vi "ARCO Instructor Write Client.vi"() -> ()   [LabVIEW 2017]
uses:
  <vilib>/OPCUA/controls/Write Status.ctl
  <vilib>/OPCUA/controls/NodeId.ctl
  <vilib>/OPCUA/client/Multiple Write Double Array.vi
  <vilib>/OPCUA/client/Multiple Write Bool Array.vi
  <vilib>/OPCUA/NI OPC UA Client.lvlib
panel:
  in  "Stop Broadcasting":bool
  in  "Time Stamp":timestamp
  in  "Node Status":T1 items=["Good"=0, "Uncertain_InitialValue"=1083310080, "Uncertain_LastUsableValue"=1083179008, "Uncertain_SensorNotAccurate"=1083375616, "Uncertain_EngineeringUnitsExceeded"=1083441152, "Bad_NoCommunication"=2150694912, "Bad_NotReadable"=2151284736, "Bad_NotWritable"=2151350272, "Bad_OutOfRange"=2151415808, "Bad_WaitingForInitialData"=2150760448]
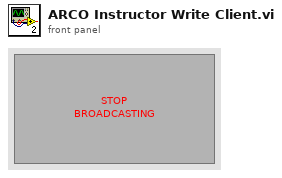
[diagram p1: front panel]
types:
  T1 = typedef "Write Status.ctl" = u32
  T2 = cluster{"message mode":enum16{"None", "Sign", "Sign and Encrypt"}, "security":enum16{"Basic256", "Basic128Rsa15"}}
  T3 = typedef "OPC UA Client Refnum.ctl" = refnum<k21>
  T4 = typedef "NodeId.ctl" = string
  T5 = cluster{"node ID":T4, "value":bool[], "timestamp (current time)":timestamp, "node status":T1}
  T6 = cluster{"node ID":T4, "value":dbl[], "timestamp (current time)":timestamp, "node status":T1}
  T7 = cluster{"node ID":T4, "value":dbl[], "timestamp (current time)":timestamp, "node status":T1}[]
  T8 = cluster{"node ID":T4, "value":bool[], "timestamp (current time)":timestamp, "node status":T1}[]
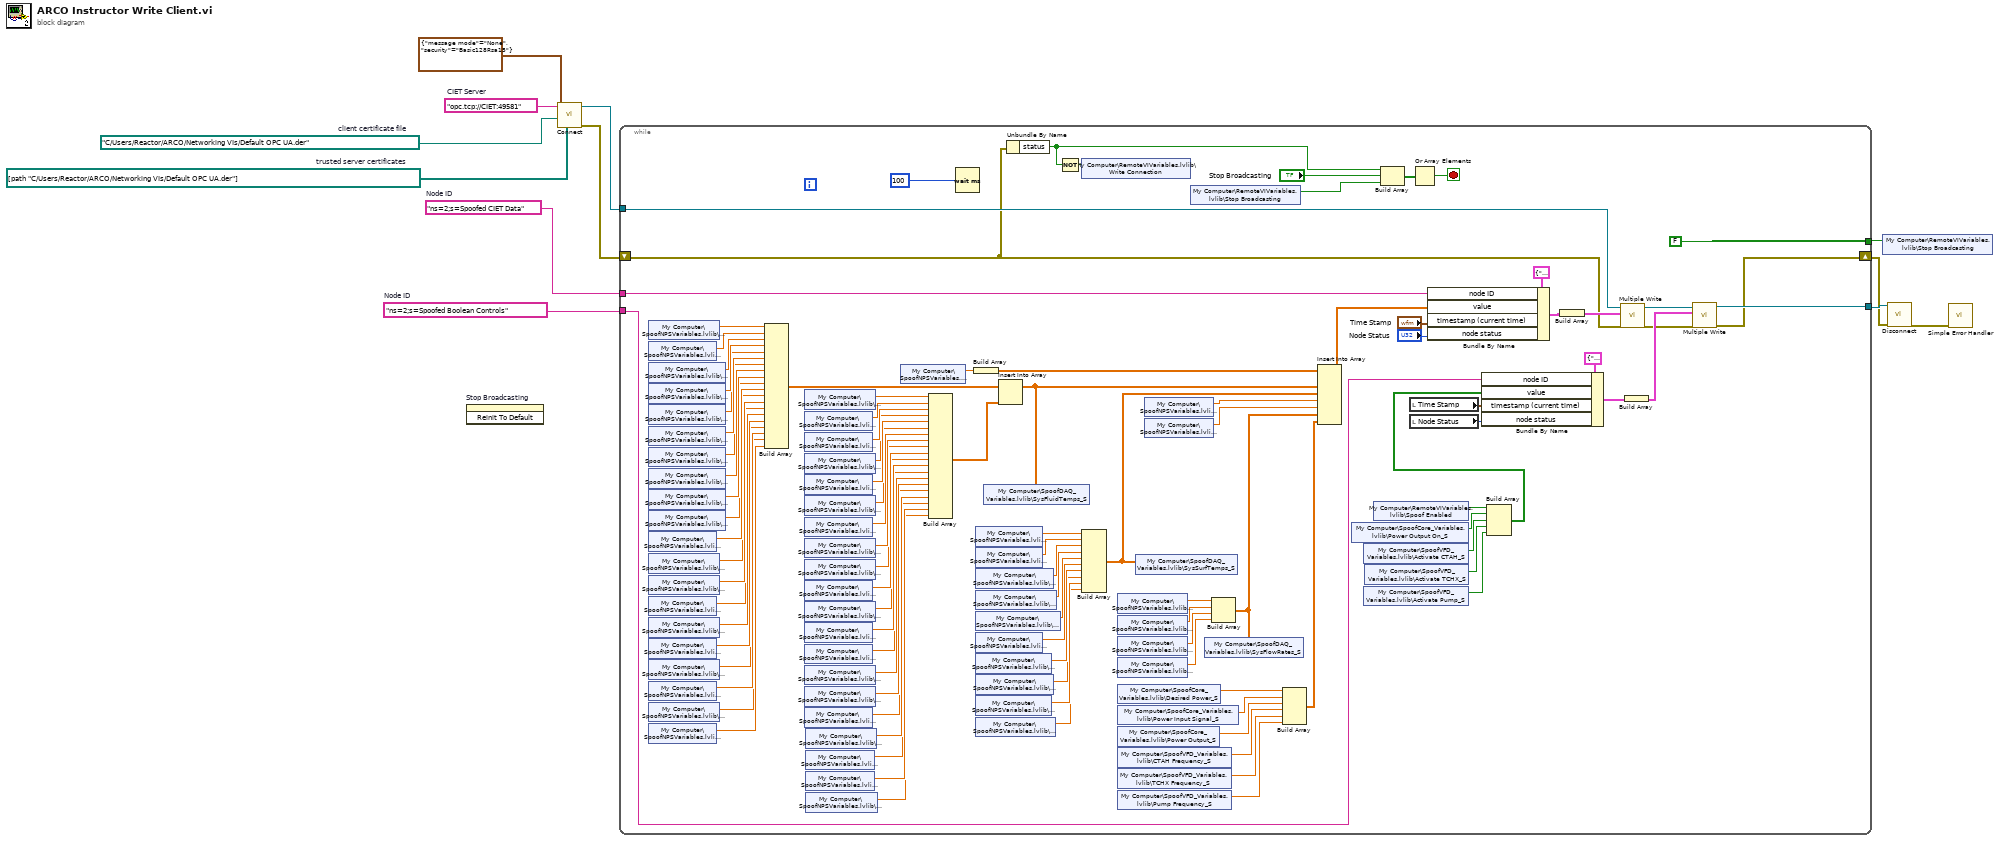
[diagram p0: block diagram]
diagram:
  w1 = "ns=2;s=Spoofed Boolean Controls"  # Node ID
  w6 = path[] [path "C:/Users/Reactor/ARCO/Networking VIs/Default OPC UA.der"]  # trusted server certificates
  w7 = path "C:/Users/Reactor/ARCO/Networking VIs/Default OPC UA.der"  # client certificate file
  w9 = "ns=2;s=Spoofed CIET Data"  # Node ID
  w11 = "opc.tcp://CIET:49581"  # CIET Server
  n1 = invoke on="Stop Broadcasting" class="Bool (strict)" method="Reinit To Default"() -> ()  [unwired: 3 in, 3 out]
  n2 = call <vilib>:"Connect.vi"("trusted server certificates"=w6, "client certificate file"=w7, "security policy"=T2 {"message mode"=enum."None", "security"=enum."Basic128Rsa15"}, "server endpoint URL"=w11) -> ("error out"=w3:errorcluster, "OPC UA client refnum out"=w10:T3)  [unwired: 5 in, 1 out]
  n3 = while {
    tunnel: w9 -> [w114]
    tunnel: w10 -> [w113]
    tunnel: [w20] -> w8
    tunnel: [FALSE] -> w4
    shift-right: [w19] -> w2
    shift-left: w3 -> [w36]
    tunnel: w1 -> [w28]
    stop <- w42 stop-if-true
    n4 = shared-variable "My Computer\\SpoofNPSVariables.lvlib\\WT-10_S"() -> (w107:sgl)  [unwired: 1 in, 1 out]
    n5 = shared-variable "My Computer\\SpoofNPSVariables.lvlib\\BT-11_S"() -> (w106:sgl)  [unwired: 1 in, 1 out]
    n6 = shared-variable "My Computer\\SpoofNPSVariables.lvlib\\CX-10-1_S"() -> (w105:sgl)  [unwired: 1 in, 1 out]
    n7 = shared-variable "My Computer\\SpoofNPSVariables.lvlib\\CX-10-2_S"() -> (w104:sgl)  [unwired: 1 in, 1 out]
    n8 = shared-variable "My Computer\\SpoofNPSVariables.lvlib\\CX-10-3_S"() -> (w103:sgl)  [unwired: 1 in, 1 out]
    n9 = shared-variable "My Computer\\SpoofNPSVariables.lvlib\\CX-10-4_S"() -> (w102:sgl)  [unwired: 1 in, 1 out]
    n10 = shared-variable "My Computer\\SpoofNPSVariables.lvlib\\CX-11-1_S"() -> (w101:sgl)  [unwired: 1 in, 1 out]
    n11 = shared-variable "My Computer\\SpoofNPSVariables.lvlib\\CX-11-2_S"() -> (w100:sgl)  [unwired: 1 in, 1 out]
    n12 = shared-variable "My Computer\\SpoofNPSVariables.lvlib\\CX-11-3_S"() -> (w99:sgl)  [unwired: 1 in, 1 out]
    n13 = shared-variable "My Computer\\SpoofNPSVariables.lvlib\\CX-11-4_S"() -> (w98:sgl)  [unwired: 1 in, 1 out]
    n14 = shared-variable "My Computer\\SpoofNPSVariables.lvlib\\BT-12_S"() -> (w97:sgl)  [unwired: 1 in, 1 out]
    n15 = shared-variable "My Computer\\SpoofNPSVariables.lvlib\\WT-13_S"() -> (w96:sgl)  [unwired: 1 in, 1 out]
    n16 = shared-variable "My Computer\\SpoofNPSVariables.lvlib\\WT-20_S"() -> (w95:sgl)  [unwired: 1 in, 1 out]
    n17 = shared-variable "My Computer\\SpoofNPSVariables.lvlib\\BT-21_S"() -> (w94:sgl)  [unwired: 1 in, 1 out]
    n18 = shared-variable "My Computer\\SpoofNPSVariables.lvlib\\WT-22_S"() -> (w93:sgl)  [unwired: 1 in, 1 out]
    n19 = shared-variable "My Computer\\SpoofNPSVariables.lvlib\\BT-23_S"() -> (w92:sgl)  [unwired: 1 in, 1 out]
    n20 = shared-variable "My Computer\\SpoofNPSVariables.lvlib\\WT-24_S"() -> (w91:sgl)  [unwired: 1 in, 1 out]
    n21 = shared-variable "My Computer\\SpoofNPSVariables.lvlib\\BT-25_S"() -> (w90:sgl)  [unwired: 1 in, 1 out]
    n22 = shared-variable "My Computer\\SpoofNPSVariables.lvlib\\WT-26_S"() -> (w89:sgl)  [unwired: 1 in, 1 out]
    n23 = shared-variable "My Computer\\SpoofNPSVariables.lvlib\\BT-27_S"() -> (w88:sgl)  [unwired: 1 in, 1 out]
    n24 = Build Array(w107, w106, w105, w104, w103, w102, w101, w100, w99, w98, w97, w96, w95, w94, w93, w92, w91, w90, w89, w88) -> (w66:sgl[])
    n25 = shared-variable "My Computer\\SpoofNPSVariables.lvlib\\WT-28_S"() -> (w87:sgl)  [unwired: 1 in, 1 out]
    n26 = shared-variable "My Computer\\SpoofNPSVariables.lvlib\\BT-29_S"() -> (w86:sgl)  [unwired: 1 in, 1 out]
    n27 = shared-variable "My Computer\\SpoofNPSVariables.lvlib\\BT-30_S"() -> (w85:sgl)  [unwired: 1 in, 1 out]
    n28 = shared-variable "My Computer\\SpoofNPSVariables.lvlib\\WT-31_S"() -> (w84:sgl)  [unwired: 1 in, 1 out]
    n29 = shared-variable "My Computer\\SpoofNPSVariables.lvlib\\BT-32_S"() -> (w83:sgl)  [unwired: 1 in, 1 out]
    n30 = shared-variable "My Computer\\SpoofNPSVariables.lvlib\\WT-33_S"() -> (w82:sgl)  [unwired: 1 in, 1 out]
    n31 = shared-variable "My Computer\\SpoofNPSVariables.lvlib\\BT-34_S"() -> (w81:sgl)  [unwired: 1 in, 1 out]
    n32 = shared-variable "My Computer\\SpoofNPSVariables.lvlib\\WT-35_S"() -> (w80:sgl)  [unwired: 1 in, 1 out]
    n33 = shared-variable "My Computer\\SpoofNPSVariables.lvlib\\WT-40_S"() -> (w79:sgl)  [unwired: 1 in, 1 out]
    n34 = shared-variable "My Computer\\SpoofNPSVariables.lvlib\\BT-41_S"() -> (w78:sgl)  [unwired: 1 in, 1 out]
    n35 = shared-variable "My Computer\\SpoofNPSVariables.lvlib\\WT-42_S"() -> (w77:sgl)  [unwired: 1 in, 1 out]
    n36 = shared-variable "My Computer\\SpoofNPSVariables.lvlib\\BT-43_S"() -> (w76:sgl)  [unwired: 1 in, 1 out]
    n37 = shared-variable "My Computer\\SpoofNPSVariables.lvlib\\BT-60_S"() -> (w75:sgl)  [unwired: 1 in, 1 out]
    n38 = shared-variable "My Computer\\SpoofNPSVariables.lvlib\\WT-61_S"() -> (w74:sgl)  [unwired: 1 in, 1 out]
    n39 = shared-variable "My Computer\\SpoofNPSVariables.lvlib\\WT-62_S"() -> (w73:sgl)  [unwired: 1 in, 1 out]
    n40 = shared-variable "My Computer\\SpoofNPSVariables.lvlib\\BT-63_S"() -> (w72:sgl)  [unwired: 1 in, 1 out]
    n41 = shared-variable "My Computer\\SpoofNPSVariables.lvlib\\WT-64_S"() -> (w71:sgl)  [unwired: 1 in, 1 out]
    n42 = shared-variable "My Computer\\SpoofNPSVariables.lvlib\\BT-65_S"() -> (w70:sgl)  [unwired: 1 in, 1 out]
    n43 = shared-variable "My Computer\\SpoofNPSVariables.lvlib\\BT-66_S"() -> (w69:sgl)  [unwired: 1 in, 1 out]
    n44 = shared-variable "My Computer\\SpoofNPSVariables.lvlib\\WT-67_S"() -> (w68:sgl)  [unwired: 1 in, 1 out]
    n45 = shared-variable "My Computer\\SpoofNPSVariables.lvlib\\Time_S"() -> (w55:sgl)  [unwired: 1 in, 1 out]
    n46 = Build Array(w87, w86, w85, w84, w83, w82, w81, w80, w79, w78, w77, w76, w75, w74, w73, w72, w71, w70, w69, w68) -> (w67:sgl[])
    n47 = Wait (ms)(milliseconds to wait=u32 100) -> ()  [unwired: 1 out]
    n48 = Build Array(w55) -> (w46:sgl[])
    n49 = shared-variable "My Computer\\SpoofNPSVariables.lvlib\\ST-10_S"() -> (w65:sgl)  [unwired: 1 in, 1 out]
    n50 = shared-variable "My Computer\\SpoofNPSVariables.lvlib\\ST-11_S"() -> (w64:sgl)  [unwired: 1 in, 1 out]
    n51 = shared-variable "My Computer\\SpoofNPSVariables.lvlib\\ST-12-N_S"() -> (w63:sgl)  [unwired: 1 in, 1 out]
    n52 = shared-variable "My Computer\\SpoofNPSVariables.lvlib\\ST-12-SE_S"() -> (w62:sgl)  [unwired: 1 in, 1 out]
    n53 = shared-variable "My Computer\\SpoofNPSVariables.lvlib\\ST-12-SW_S"() -> (w61:sgl)  [unwired: 1 in, 1 out]
    n54 = shared-variable "My Computer\\SpoofNPSVariables.lvlib\\ST-13_S"() -> (w60:sgl)  [unwired: 1 in, 1 out]
    n55 = shared-variable "My Computer\\SpoofNPSVariables.lvlib\\ST-14-E_S"() -> (w59:sgl)  [unwired: 1 in, 1 out]
    n56 = shared-variable "My Computer\\SpoofNPSVariables.lvlib\\ST-14-N_S"() -> (w58:sgl)  [unwired: 1 in, 1 out]
    n57 = shared-variable "My Computer\\SpoofNPSVariables.lvlib\\ST-14-S_S"() -> (w57:sgl)  [unwired: 1 in, 1 out]
    n58 = shared-variable "My Computer\\SpoofNPSVariables.lvlib\\ST-14-W_S"() -> (w56:sgl)  [unwired: 1 in, 1 out]
    n59 = Insert Into Array(array=w66, new element=w67) -> (w54:sgl[])  [unwired: 1 in]
    n60 = shared-variable "My Computer\\SpoofDAQ_Variables.lvlib\\SysFluidTemps_S"(w54) -> ()  [unwired: 1 in, 1 out]
    n61 = Unbundle By Name(w36) -> ("status"=w38:bool)
    n62 = Not(x=w38) -> (.not. x?=w37:bool)
    n63 = shared-variable "My Computer\\RemoteVIVariables.lvlib\\Write Connection"(w37) -> ()  [unwired: 1 in, 1 out]
    n64 = Build Array(w65, w64, w63, w62, w61, w60, w59, w58, w57, w56) -> (w45:sgl[])
    n65 = shared-variable "My Computer\\SpoofNPSVariables.lvlib\\FM-20_S"() -> (w51:sgl)  [unwired: 1 in, 1 out]
    n66 = shared-variable "My Computer\\SpoofNPSVariables.lvlib\\FM-30_S"() -> (w50:sgl)  [unwired: 1 in, 1 out]
    n67 = shared-variable "My Computer\\SpoofNPSVariables.lvlib\\FM-40_S"() -> (w49:sgl)  [unwired: 1 in, 1 out]
    n68 = shared-variable "My Computer\\SpoofNPSVariables.lvlib\\FM-60_S"() -> (w48:sgl)  [unwired: 1 in, 1 out]
    n69 = shared-variable "My Computer\\SpoofCore_Variables.lvlib\\Desired Power_S"() -> (w35:sgl)  [unwired: 1 in, 1 out]
    n70 = shared-variable "My Computer\\SpoofCore_Variables.lvlib\\Power Input Signal_S"() -> (w34:sgl)  [unwired: 1 in, 1 out]
    n71 = shared-variable "My Computer\\SpoofCore_Variables.lvlib\\Power Output_S"() -> (w33:sgl)  [unwired: 1 in, 1 out]
    n72 = shared-variable "My Computer\\SpoofVFD_Variables.lvlib\\CTAH Frequency_S"() -> (w32:sgl)  [unwired: 1 in, 1 out]
    n73 = shared-variable "My Computer\\SpoofVFD_Variables.lvlib\\TCHX Frequency_S"() -> (w31:sgl)  [unwired: 1 in, 1 out]
    n74 = shared-variable "My Computer\\SpoofVFD_Variables.lvlib\\Pump Frequency_S"() -> (w30:sgl)  [unwired: 1 in, 1 out]
    n75 = shared-variable "My Computer\\SpoofDAQ_Variables.lvlib\\SysSurfTemps_S"(w45) -> ()  [unwired: 1 in, 1 out]
    n76 = shared-variable "My Computer\\SpoofNPSVariables.lvlib\\AT-01_S"() -> (w53:sgl)  [unwired: 1 in, 1 out]
    n77 = shared-variable "My Computer\\SpoofNPSVariables.lvlib\\AT-02_S"() -> (w52:sgl)  [unwired: 1 in, 1 out]
    n78 = shared-variable "My Computer\\RemoteVIVariables.lvlib\\Stop Broadcasting"() -> (w40:bool)  [unwired: 1 in, 1 out]
    n79 = Build Array(w51, w50, w49, w48) -> (w47:sgl[])
    n80 = shared-variable "My Computer\\SpoofDAQ_Variables.lvlib\\SysFlowRates_S"(w47) -> ()  [unwired: 1 in, 1 out]
    n81 = Build Array(w35, w34, w33, w32, w31, w30) -> (w29:sgl[])
    n82 = Insert Into Array(array=w46, new element #1=w54, new element #2=w45, new element #3=w53, new element #4=w52, new element #5=w47, new element #6=w29) -> (w44:sgl[])  [unwired: 1 in]
    n83 = shared-variable "My Computer\\SpoofCore_Variables.lvlib\\Power Output On_S"() -> (w16:bool)  [unwired: 1 in, 1 out]
    n84 = shared-variable "My Computer\\SpoofVFD_Variables.lvlib\\Activate CTAH_S"() -> (w15:bool)  [unwired: 1 in, 1 out]
    n85 = shared-variable "My Computer\\SpoofVFD_Variables.lvlib\\Activate Pump_S"() -> (w13:bool)  [unwired: 1 in, 1 out]
    n86 = shared-variable "My Computer\\SpoofVFD_Variables.lvlib\\Activate TCHX_S"() -> (w14:bool)  [unwired: 1 in, 1 out]
    n87 = shared-variable "My Computer\\RemoteVIVariables.lvlib\\Spoof Enabled"() -> (w26:bool)  [unwired: 1 in, 1 out]
    n88 = Build Array(w38, "Stop Broadcasting", w40) -> (w41:bool[])
    n89 = local read "Time Stamp"() -> (w18:timestamp)
    n90 = local read "Node Status"() -> (w17:T1)
    n91 = Or Array Elements(Boolean array=w41) -> (logical OR=w42:bool)
    n92 = Bundle By Name(cluster=T6 {"node ID"="", "value"=[], "timestamp (current time)"=timestamp(0 s since 1904-01-01), "node status"=0} ("request"), "node ID"=w114, "value"=w44, "timestamp (current time)"="Time Stamp", "node status"="Node Status") -> (w109:T6)
    n93 = Build Array(w26, w16, w15, w14, w13) -> (w25:bool[])
    n94 = Bundle By Name(cluster=T5 {"node ID"="", "value"=[], "timestamp (current time)"=timestamp(0 s since 1904-01-01), "node status"=0} ("request"), "node ID"=w28, "value"=w25, "timestamp (current time)"=w18, "node status"=w17) -> (w24:T5)
    n95 = Build Array(w109) -> (w108:T7)
    n96 = call-poly <vilib>:"Multiple Write.vi"("error in (no error)"=w36, "requests"=w108, "OPC UA client refnum in"=w113) -> ("error out"=w21:errorcluster, "OPC UA client refnum out"=w22:T3)  [unwired: 5 in, 2 out]
    n97 = Build Array(w24) -> (w23:T8)
    n98 = call-poly <vilib>:"Multiple Write.vi"("error in (no error)"=w21, "requests"=w23, "OPC UA client refnum in"=w22) -> ("error out"=w19:errorcluster, "OPC UA client refnum out"=w20:T3)  [unwired: 5 in, 2 out]
  }
  n99 = shared-variable "My Computer\\RemoteVIVariables.lvlib\\Stop Broadcasting"(w4) -> ()  [unwired: 1 in, 1 out]
  n100 = call <vilib>:"Disconnect.vi"("error in (no error)"=w2, "OPC UA client refnum in"=w8) -> ("error out"=w12:errorcluster)  [unwired: 9 in]
  n101 = call <vilib>:"Simple Error Handler.vi"("error in (no error)"=w12) -> ()  [unwired: 4 in, 5 out]
